vi "Vector_Dilatation.vi"(8 "error in":errorcluster caption="entrée d'erreur", 10 "# of duplication":u16=1 min=1, 11 "Vecteur in":dbl[](array[numeric])) -> (0 "error out":errorcluster caption="sortie d'erreur", 3 "Duplicated vector":dbl[](array[numeric]))   [LabVIEW 2026]
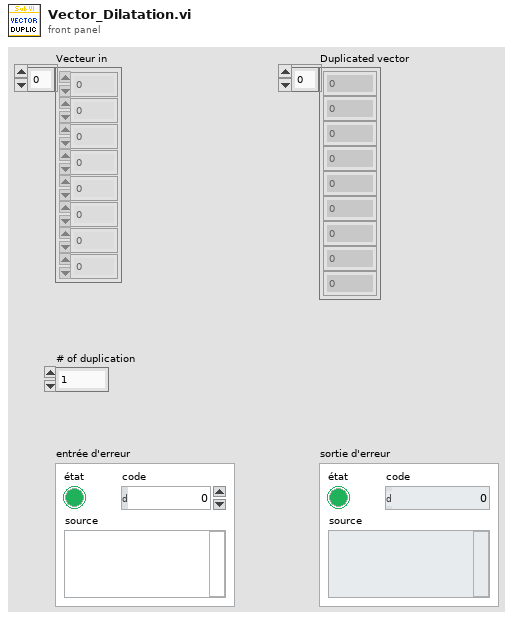
[diagram p1: front panel]
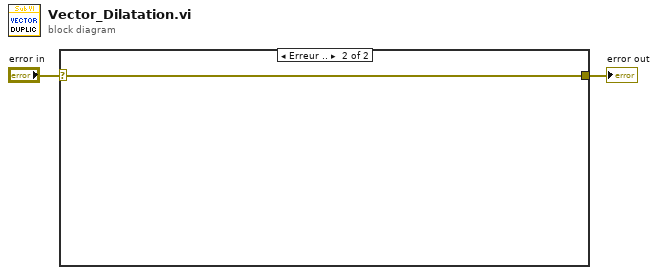
[diagram p0: block diagram]
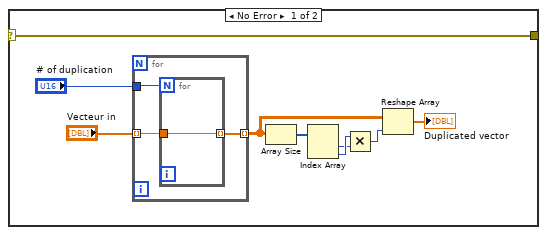
[diagram p2: hidden frame]
diagram:
  n1 = case shown="Erreur .." "error in" {
    selector: "error in" -> [w3 w16]
    tunnel: [w3 w16] -> w1
    frame No Error {
      n2 = for {
        tunnel: "# of duplication" -> [w13]
        tunnel: "Vecteur in" -> [w14] mode=indexing
        tunnel: [w12] -> w7 mode=indexing
        n3 = for {
          N: w13 -> [_]
          tunnel: w14 -> [w15]
          tunnel: [w15] -> w12 mode=indexing
        }
      }
      n4 = Array Size(array=w7) -> (size(s)=w8:i32[])
      n5 = Index Array(array=w8) -> (element #1=w9:i32, element #2=w10:i32)  [unwired: 2 in]
      n6 = Multiply(x=w10, y=w9) -> (x*y=w11:i32)
      n7 = Reshape Array(w7, w11) -> (→"Duplicated vector":dbl[])
    }
    frame Error {
    }
  }
  "error out" <- w1
